vi "readFromXML.vi"(8 "error in (no error)":errorcluster, 10 "XMLin":string="<AzElParameters>\n  <azimuth>\n    <degreesArc>44.33</degreesArc>\n    <minutesArc>33.22</minutesArc>\n    <secondsArc>22.11</secondsArc>\n  </azimuth>\n  <elevation>\n    <degreesAlt>90.20</degreesAlt>\n    <minutesArc>80.30</minutesArc>\n    <secondsArc>70.40</secondsArc>\n  </elevation>\n</AzElParameters>", 11 "AzElParameters in":refnum<class "AzElParameters.lvclass">) -> (0 "error out":errorcluster, 3 "AzElParameters out":refnum<class "AzElParameters.lvclass">)   [LabVIEW 2014, in "TCSDataDefinitions.lvlib" / "TCSCommand.lvlib" / "TargetConfiguration.lvlib" / "Target.lvlib" / "FixedTarget.lvlib" / "AzElParameters.lvclass"]
uses:
  AzElParameters.lvclass
  Azimuth/Azimuth.lvclass
  Elevation/Elevation.lvclass
  AzElParameters.lvclass/AzElParameters.ctl
  <userlib>/Common/XML/XMLParser/XMLParser.lvclass
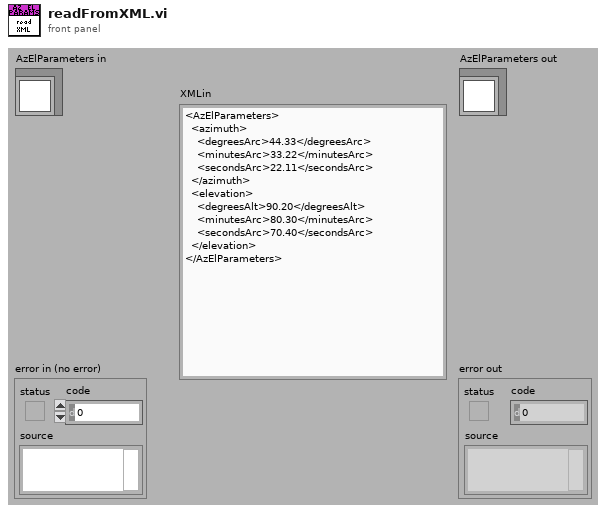
[diagram p1: front panel]
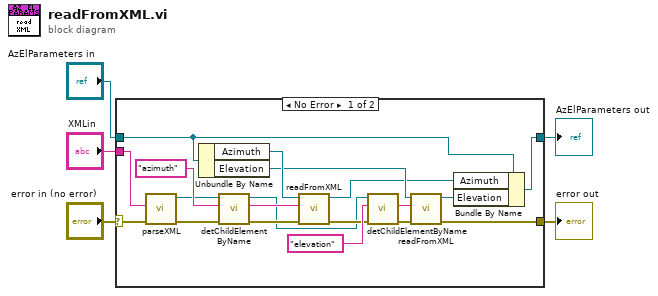
[diagram p0: block diagram]
diagram:
  n1 = case shown="No Error" "error in (no error)" {
    selector: "error in (no error)" -> [w9 w26]
    tunnel: [w8 w26] -> w4
    tunnel: [w22 w25] -> w2
    tunnel: "AzElParameters in" -> [w23 w25]
    tunnel: "XMLin" -> [w24 _]
    frame No Error {
      n2 = call <userlib>:"parseXML.vi"("error in (no error)"=w9, "XMLString in"=w24) -> ("error out"=w19:errorcluster, "Element out"=w7:refnum<class "XMLParser.lvclass">)  [unwired: 8 in]
      n3 = Unbundle By Name(w23) -> ("Azimuth"=w17:refnum<class "Azimuth.lvclass">, "Elevation"=w16:refnum<class "Elevation.lvclass">)
      n4 = call <userlib>:"detChildElementByName.vi"("error in (no error)"=w19, "childName"="azimuth" ("ChildName"), "Element in"=w7) -> ("error out"=w20:errorcluster, "childXML"=w18:string, "Element out"=w6:refnum<class "XMLParser.lvclass">)  [unwired: 5 in, 1 out]
      n5 = call-dynamic "readFromXML.vi"("error in (no error)"=w20, "XML in"=w18, "Azimuth in"=w17) -> ("error out"=w10:errorcluster, "Azimuth out"=w14:refnum<class "Azimuth.lvclass">)  [unwired: 7 in]
      n6 = call <userlib>:"detChildElementByName.vi"("error in (no error)"=w10, "childName"="elevation" ("ChildName"), "Element in"=w6) -> ("error out"=w11:errorcluster, "childXML"=w12:string)  [unwired: 5 in, 2 out]
      n7 = call-dynamic "readFromXML.vi"("error in (no error)"=w11, "XML in"=w12, "Elevation in"=w16) -> ("error out"=w8:errorcluster, "Elevation out"=w15:refnum<class "Elevation.lvclass">)  [unwired: 7 in]
      n8 = Bundle By Name(cluster=w23, "Azimuth"=w14, "Elevation"=w15) -> (w22:refnum<class "AzElParameters.lvclass">)
    }
    frame Error {
    }
  }
  "error out" <- w4
  "AzElParameters out" <- w2
